vi "recover it.vi"   [LabVIEW 2009]
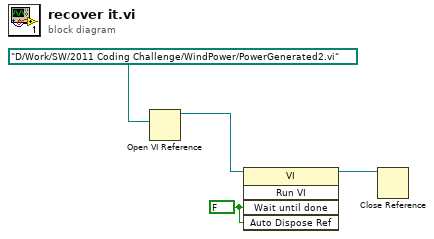
[diagram p0: block diagram]
diagram:
  w2 = FALSE ("Wait Until Done")
  n1 = Open VI Reference(vi path=path "D:/Work/SW/2011 Coding Challenge/WindPower/PowerGenerated2.vi") -> (vi reference=w3:refnum<vi>)  [unwired: 5 in, 1 out]
  n2 = invoke class="VI" method="Run VI"(reference=w3, "Wait until done"=w2, "Auto Dispose Ref"=w2) -> (reference out=w1:refnum<vi>)  [unwired: 2 in, 4 out]
  n3 = Close Reference(reference=w1) -> ()  [unwired: 1 in, 1 out]
